vi "Set Default.vi"(8 "error in (no error)":errorcluster, 11 "Reorder Driver Aliases Msg in":refnum<class "Reorder Driver Aliases Msg.lvclass">) -> (0 "error out":errorcluster, 3 "Reorder Driver Aliases Msg out":refnum<class "Reorder Driver Aliases Msg.lvclass">)   [LabVIEW 2020, in "Instrument Handler.lvlib" / "Reorder Driver Aliases Msg.lvclass"]
doc: "Restore private data to a defined default state.\n\nThis implementation sets:\nPublish = FALSE\nAwait Reply with -1ms Timeout\nPriority = High"
uses:
  Reorder Driver Aliases Msg.lvclass
  C:/Current projects/WS/Framework/Framework/Actors/Instrument Handler/Instrument Handler Messages/Instrument Handler Response Msg/Instrument Handler Response Msg.lvclass
  PPL/HDH.Actor Framework.Core.Publisher.lvlibp/Messages/Response Msg/Response Core/Controls/Ctl_SendFunction.ctl
  PPL/HDH.Actor Framework.Core.Actor.lvlibp/1abvi3w/vi.lib/ActorFramework/Message Enqueuer/Message Priority.ctl
  Instrument Handler Response Msg/Instrument Handler Response Msg.lvclass/Instrument Handler Response Msg.ctl
  Instrument Handler Response Msg/Instrument Handler Response Msg.lvclass
  PPL/HDH.Actor Framework.Core.Publisher.lvlibp
  PPL/HDH.Actor Framework.Core.Actor.lvlibp/1abvi3w/vi.lib/ActorFramework/Message Enqueuer/Message Enqueuer.lvclass
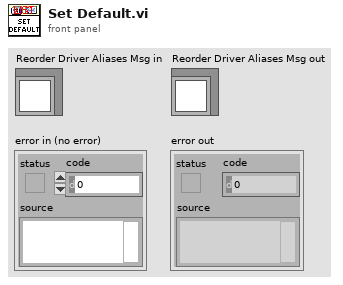
[diagram p1: front panel]
types:
  T1 = typedef "HDH.Actor Framework.Core.Actor.lvlibp/Message Enqueuer.lvclass/Message Priority.ctl" = enum16{"Low", "Normal", "High"}
  T2 = typedef "HDH.Actor Framework.Core.Publisher.lvlibp/Ctl_SendFunction.ctl" = enum16{"Send and Forget", "Request Reply", "Await Reply"}
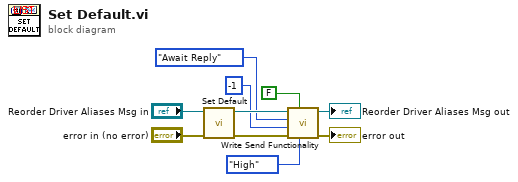
[diagram p0: block diagram]
diagram:
  n1 = call-parent "Set Default.vi"("error in (no error)"="error in (no error)", "Flex Msg in"="Reorder Driver Aliases Msg in") -> ("error out"=w6:errorcluster, "Flex Msg out"=w8:refnum<class "Reorder Driver Aliases Msg.lvclass">)  [unwired: 8 in]
  n2 = call "Write Send Functionality.vi"("Message Priority"=Message_Priority."High", "Publish Data?(T)"=FALSE, "error in (no error)"=w6, "Timeout if Waiting(-1ms)"=-1, "Send Function(Await Reply)"=Ctl_SendFunction."Await Reply", "Instrument Handler Reponse Msg in"=w8) -> ("error out"=→"error out":errorcluster, "Instrument Handler Reponse Msg out"=→"Reorder Driver Aliases Msg out":refnum<class "Reorder Driver Aliases Msg.lvclass">)  [unwired: 4 in]
